vi "WPI_CameraGet Image.vi"(8 "error in (no error)":errorcluster, 10 "Image":T1, 11 "CameraDevRef":T2={"Camera Address"="192.168.0.90", "CameraStatus"={"status"=FALSE, "code"=0, "source"=""}}) -> (0 "error out":errorcluster, 2 "Image Out":T1, 3 "CameraDevRef Out":T2)   [LabVIEW 2017]
doc: "Retrieves a specific image from the image data that the camera you specify acquired. Use the Start VI to start acquiring image data from the camera before you use the Get Image VI to retrieve an image. When you run this VI, this VI retrieves the most current snapshot of the image data from the camera.\n\nThis software is licensed. Open the labview\\readme\\WPI Robotics Library Open Source License.txt file for more information."
uses:
  <vilib>/Rock Robotics/WPI/Camera/WPI_CameraDevRef.ctl
  <vilib>/vision/Image Controls.llb/IMAQ Image.ctl
  <vilib>/picture/picture.llb/imagedata.ctl
  <vilib>/vision/driver/NI_Vision_Acquisition_Software.lvlib
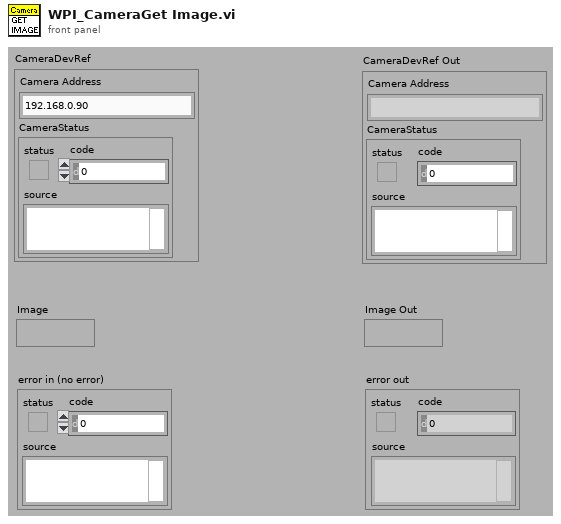
[diagram p1: front panel]
types:
  T1 = typedef "IMAQ Image.ctl" = refnum<image>
  T2 = typedef "WPI_CameraDevRef.ctl" = cluster{"Camera Address":string, "CameraStatus":errorcluster}
  T3 = typedef "imagedata.ctl" = cluster{"image type":i32, "image depth":i32, "image":u8[], "mask":u8[], "colors":u32[], "Rectangle":cluster{"left":i16, "top":i16, "right":i16, "bottom":i16}}
  T4 = typedef "WPI_CameraFrameRate.ctl" = u32
  T5 = typedef "IMAQdx.ctl" = refnum<k21>
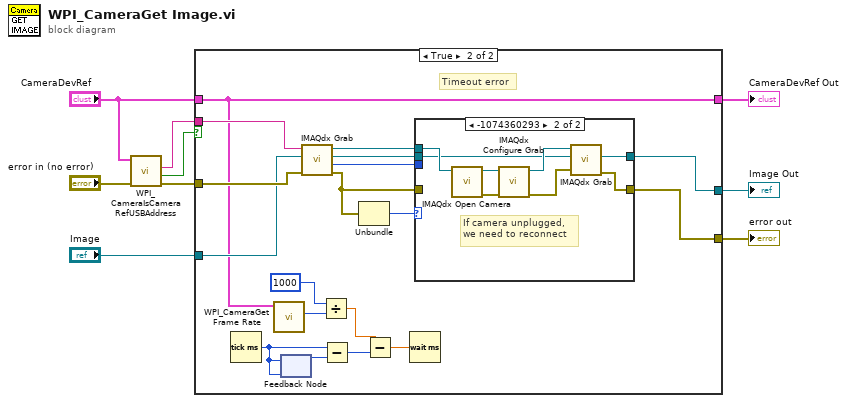
[diagram p0: block diagram]
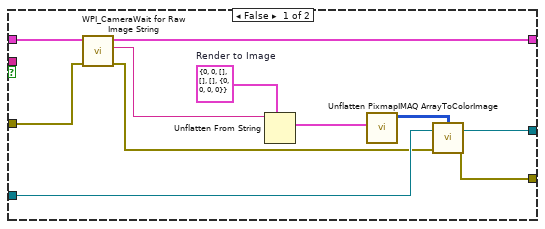
[diagram p2: hidden frame]
diagram:
  n1 = call <vilib>:"WPI_CameraIsCameraRefUSBAddress.vi"("error in (no error)"="error in (no error)", "CameraDevRef"="CameraDevRef") -> ("error out"=w3:errorcluster, "USB?"=w1:bool, "Camera Address Out"=w2:string)  [unwired: 6 in, 1 out]
  n2 = case shown="True" w1 {
    tunnel: [w20 w27] -> w9
    tunnel: w3 -> [w19 w37]
    tunnel: "CameraDevRef" -> [w18 w27]
    tunnel: "Image" -> [w17 w36]
    tunnel: [w16 w35] -> w7
    tunnel: [w15 w33] -> w6
    tunnel: w2 -> [_ w38]
    frame False {
      w12 = T3 {"image type"=0, "image depth"=0, "image"=[], "mask"=[], "colors"=[], "Rectangle"={"left"=0, "top"=0, "right"=0, "bottom"=0}}  # Render to Image
      n3 = call <vilib>:"WPI_CameraWait for Raw Image String.vi"("error in (no error)"=w19, "CameraDevRef"=w18) -> ("error out"=w11:errorcluster, "String"=w10:string, "CameraDevRef Out"=w20:T2)  [unwired: 3 in, 4 out]
      n4 = Unflatten From String(type=w12, binary string=w10) -> (value=w13:T3)  [unwired: 3 in, 2 out]
      n5 = call <vilib>:"Unflatten Pixmap.vi"("image data"=w13) -> ("24-bit pixmap"=w14:u32[][])  [unwired: 4 in, 6 out]
      n6 = call "IMAQ ArrayToColorImage"("Image Pixels (U32)"=w14, "Image"=w17, "error in (no error)"=w11) -> ("Image Out"=w15:T1, "error out"=w16:errorcluster)  [unwired: 2 in]
    }
    frame True {
      # "Timeout error"
      n7 = Tick Count (ms)() -> (millisecond timer value=w21:u32)
      n8 = call <vilib>:"WPI_CameraGet Frame Rate.vi"("CameraDevRef"=w27) -> ("Frame Rate (fps)"=w25:T4)  [unwired: 8 in, 2 out]
      n9 = feedback-in #1(w21) -> ()
      n10 = feedback #1(w21) -> (w28:u32)
      n11 = call <vilib>:"IMAQdx Grab.vi"("error in"=w37, "Image In"=w36, "Session In"=w38) -> ("error out"=w29:errorcluster, "Buffer Number Out"=w32:u32, "Image Out"=w34:T1, "Session Out"=w31:T5)  [unwired: 5 in]
      n12 = Divide(x=1000, y=w25) -> (x/y=w23:dbl)
      n13 = Subtract(x=w21, y=w28) -> (x-y=w24:u32)
      n14 = Unbundle(w29) -> ("code"=w30:i32)  [unwired: 2 out]
      n15 = Subtract(x=w23, y=w24) -> (x-y=w22:dbl)
      n16 = Wait (ms)(milliseconds to wait=w22) -> ()  [unwired: 1 out]
      n17 = case shown="-1074360293" w30 {
        tunnel: [w39 w46] -> w35
        tunnel: w34 -> [w40 w41]
        tunnel: [w40 w42] -> w33
        tunnel: w32 -> [_ _]
        tunnel: w31 -> [_ w45]
        tunnel: w29 -> [w39 _]
        frame 0, Default {
        }
        frame -1074360293 {
          # "If camera unplugged,\nwe need to reconnect"
          n18 = call <vilib>:"IMAQdx Open Camera.vi"("Session In"=w45) -> ("error out"=w48:errorcluster, "Session Out"=w44:T5)  [unwired: 9 in]
          n19 = call <vilib>:"IMAQdx Configure Grab.vi"("error in"=w48, "Session In"=w44) -> ("error out"=w47:errorcluster, "Session Out"=w43:T5)  [unwired: 8 in]
          n20 = call <vilib>:"IMAQdx Grab.vi"("error in"=w47, "Image In"=w41, "Session In"=w43) -> ("error out"=w46:errorcluster, "Image Out"=w42:T1)  [unwired: 5 in, 2 out]
        }
      }
    }
  }
  "CameraDevRef Out" <- w9
  "Image Out" <- w6
  "error out" <- w7
